vi "Configure Measurement Signal.vi"(0 "reference in":refnum<class "BKP-891 LCR Meter.lvclass">, 1 "Signal Frequency (1000 Hz)":dbl=1000.0 format="%#_4g", 2 "Signal Level (0:0.5 Vrms)":u8(ring) items=["0.5Vrms", "1Vrms"], 5 "error in (no error)":errorcluster) -> (14 "reference out":refnum<class "BKP-891 LCR Meter.lvclass">, 19 "error out":errorcluster)   [LabVIEW 2018, in "BKP-891 LCR Meter.lvclass"]
uses:
  BKP-891 LCR Meter.lvclass
  <instrlib>/BK Precision 891/BK Precision 891.lvlib
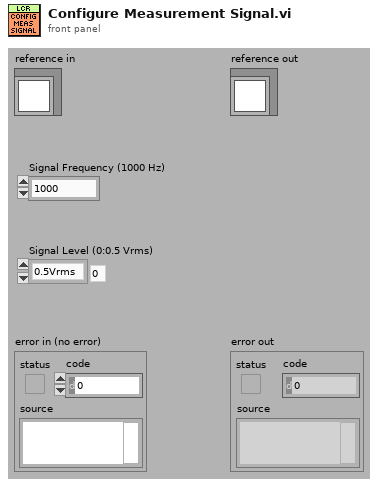
[diagram p1: front panel]
types:
  T1 = typedef "BKP-891 LCR Meter.lvclass/ObjectAttributes.ctl" = cluster{"VISA resource name":refnum<visa-resource-name>, "Simulated?":bool, "Latest Values":dbl[], "Signal List":T2[], "Tare Offset":dbl[], "Range":u16, "Measurement Speed":u16, "Function":u16, "Signal Frequency (Hz)":dbl, "Signal Level (Vrms)":u8, "UVW Mode":enum16{"UV", "UW", "VW", "None"}, "LR Mode":T3, "Primary Parameter":string, "Secondary Parameter":string}
  T2 = typedef "IO Signal List.ctl" = enum16{"Timestamp", "PSU_FB_U_VDC", "PSU_FB_I_AMP", "PSU_FB_W_WATT", "PSU_CMD_U_VDC", "PSU_CMD_I_AMP", "PSU_CMD_OUTPUT", "LCR_PRIMARY", "LCR_SECONDARY", "UV_R_Ohm", "UW_R_Ohm", "VW_R_Ohm", "UV_L_H", "UW_L_H", "VW_L_H", "U_U_VDC", "V_U_VDC", "W_U_VDC", "U_I_AMP", "V_I_AMP", "W_I_AMP", "PWM_CMD_DC_%", "PWM_CMD_VDC", "PWM_CMD_Hz", "PWM_FB_DC_%", "PWM_FB_VDC", "PWM_FB_Hz", "DO_RELAY_U_LCR_A", "DO_RELAY_V_LCR_A", "DO_RELAY_V_LCR_B", "DO_RELAY_W_LCR_B", "DIFF_UV_UW_L_H", "DIFF_UV_VW_L_H", "DIFF_UW_VW_L_H", "DIFF_UV_UW_R_Ohm", "DIFF_UV_VW_R_Ohm", "DIFF_UW_VW_R_Ohm", "DIFF_UV_U_VDC", "DIFF_UW_U_VDC", "DIFF_VW_U_VDC"}
  T3 = typedef "LR Mode.ctl" = enum16{"R - Resistance", "L - Inductance"}
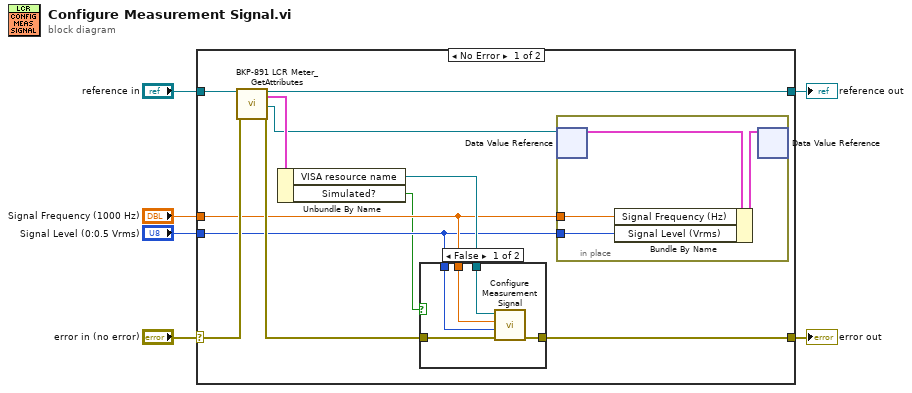
[diagram p0: block diagram]
diagram:
  n1 = case shown="No Error" "error in (no error)" {
    selector: "error in (no error)" -> [w17 w29]
    tunnel: [w12 w29] -> w5
    tunnel: [w14 w28] -> w3
    tunnel: "reference in" -> [w15 w28]
    tunnel: "Signal Frequency (1000 Hz)" -> [w9 _]
    tunnel: "Signal Level (0:0.5 Vrms)" -> [w8 _]
    frame No Error {
      n2 = call "BKP-891 LCR Meter_GetAttributes.vi"("reference in"=w15, "error in (no error)"=w17) -> ("reference out"=w14:refnum<class "BKP-891 LCR Meter.lvclass">, "Data"=w16:T1, "DataRef"=w10:refnum<data-value>, "error out"=w13:errorcluster)  [unwired: 14 in]
      n3 = Unbundle By Name(w16) -> ("VISA resource name"=w11:refnum<visa-resource-name>, "Simulated?"=w7:bool)
      n4 = case shown="False" w7 {
        tunnel: w13 -> [w22 w23]
        tunnel: [w21 w23] -> w12
        tunnel: w11 -> [w20 _]
        tunnel: w9 -> [w19 _]
        tunnel: w8 -> [w18 _]
        frame False {
          n5 = call <instrlib>:"Configure Measurement Signal.vi"("error in (no error)"=w22, "Signal Level (0:0.5 Vrms)"=w18, "Signal Frequency (1000 Hz)"=w19, "VISA resource name"=w20) -> ("error out"=w21:errorcluster)  [unwired: 6 in, 1 out]
        }
        frame True {
        }
      }
      n6 = in-place {
        in-place-border: w9 -> [w25]
        in-place-border: w8 -> [w24]
        n7 = in-place-dvr #1(w10) -> (w27:T1)  [unwired: 1 out]
        n8 = Bundle By Name(cluster=w27, "Signal Frequency (Hz)"=w25, "Signal Level (Vrms)"=w24) -> (w26:T1)
        n9 = in-place-dvr #1(w26) -> ()  [unwired: 2 out]
      }
    }
    frame Error {
    }
  }
  "error out" <- w5
  "reference out" <- w3
